vi "movearea_old.vi"(8 "error in (no error)":errorcluster, 11 "Input":string="y-") -> (0 "error out":errorcluster, 3 "Output":string)   [LabVIEW 2014]
uses:
  <userlib>/Nanonis Prog Interface V5/Nanonis Prog Interface.lvlib
panel:
  out "size(s)":i32=3
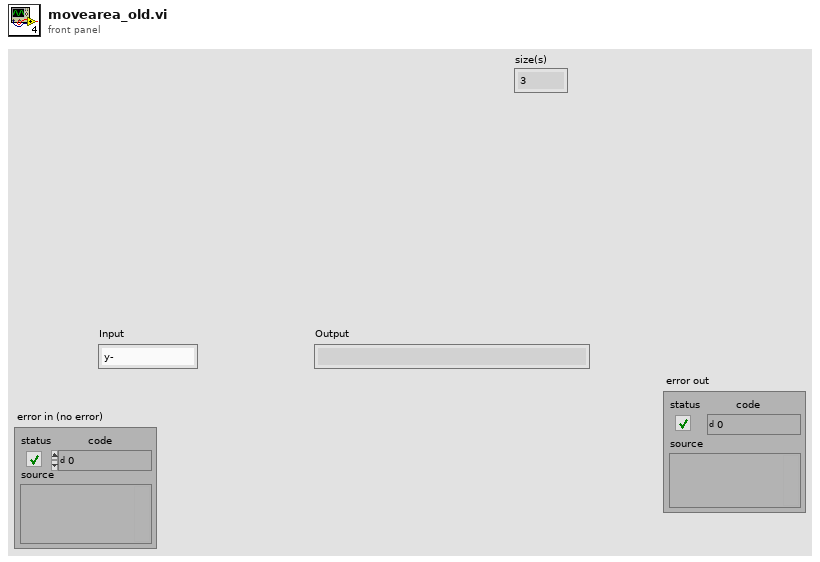
[diagram p1: front panel]
types:
  T1 = enum8{"Group 1", "Group 2", "Group 3", "Group 4", "Group 5", "Group 6"}
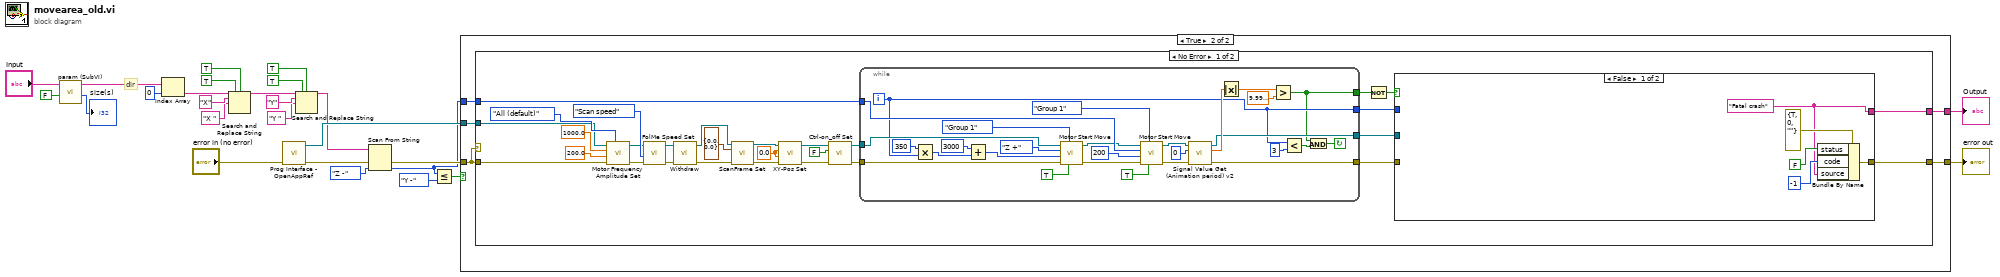
[diagram p0: block diagram]
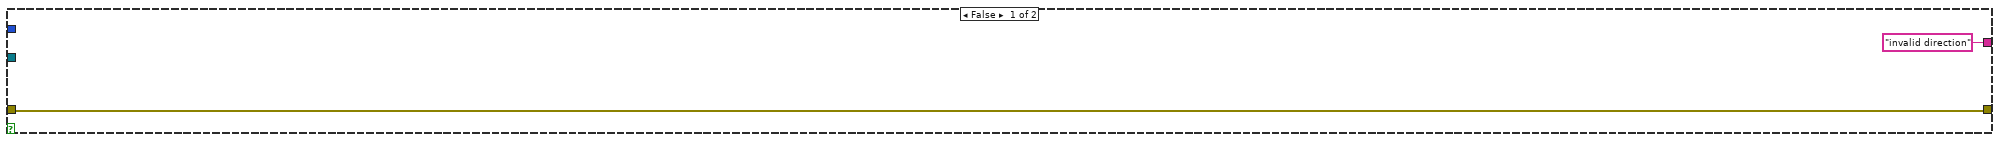
[diagram p2: hidden frame]
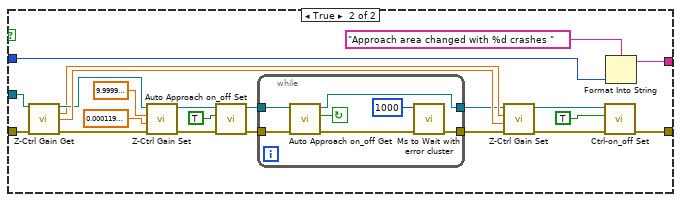
[diagram p3: hidden frame]
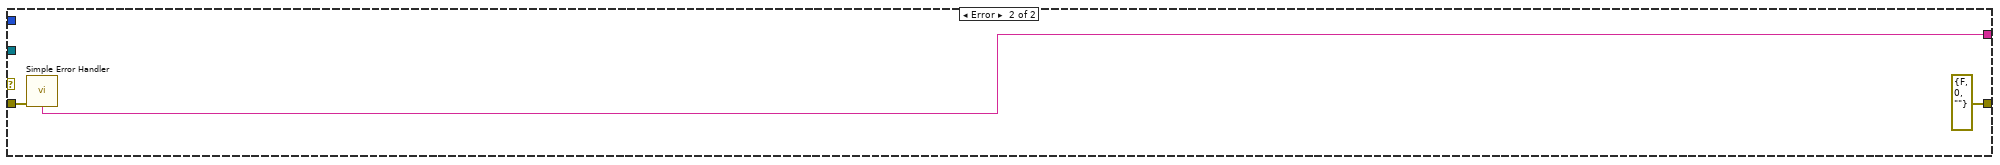
[diagram p4: hidden frame]
diagram:
  # "dir"
  n1 = call <userlib>:"param (SubVI).vi"("Numeric"=FALSE, "Input"="Input") -> ("num"=→"size(s)":i32, "Array"=w22:string[])  [unwired: 7 in, 1 out]
  n2 = Index Array(array=w22, index=0) -> (element=w11:string)
  n3 = Search and Replace String(replace all?=TRUE ("replace all? (F)"), case sensitive?=TRUE ("ignore case? (F)"), input string=w11, search string="X", replace string="X " ("replace string (\"\")")) -> (result string=w2:string)  [unwired: 3 in, 3 out]
  n4 = call <userlib>:"Prog Interface - OpenAppRef.vi"("Error in (no error)"="error in (no error)") -> ("Error out"=w19:errorcluster, "Application reference"=w23:refnum<vi>)  [unwired: 5 in]
  n5 = Search and Replace String(replace all?=TRUE ("replace all? (F)"), case sensitive?=TRUE ("ignore case? (F)"), input string=w2, search string="Y", replace string="Y " ("replace string (\"\")")) -> (result string=w1:string)  [unwired: 3 in, 3 out]
  n6 = Scan From String(input string=w1, error in=w19, default 1=enum16{"X +", "X -", "Y +", "Y -", "Z +", "Z -"}."Z -" ("Direction")) -> (error out=w18:errorcluster, output 1=w15:enum16{"X +", "X -", "Y +", "Y -", "Z +", "Z -"})  [unwired: 2 in, 2 out]
  n7 = Less Or Equal?(x=w15, y=enum16{"X +", "X -", "Y +", "Y -", "Z +", "Z -"}."Y -") -> (x <= y?=w13:bool)
  n8 = case shown="True" w13 {
    tunnel: w23 -> [_ w33]
    tunnel: w15 -> [_ w32]
    tunnel: w18 -> [w28 w31]
    tunnel: [w28 w30] -> w17
    tunnel: ["invalid direction" ("message") w29] -> w16
    frame False {
    }
    frame True {
      n9 = case shown="No Error" w31 {
        tunnel: w33 -> [w50 _]
        tunnel: w32 -> [w48 _]
        tunnel: w31 -> [w47 w127]
        tunnel: [w34 errorcluster {"status"=FALSE, "code"=0, "source"=""} ("error out")] -> w30
        tunnel: [w39 w126] -> w29
        frame No Error {
          w57 = sgl 0.0 ("X (m)")
          n10 = call <userlib>:"Motor Frequency Amplitude Set.vi"("Axis (All)"=enum16{"All (default)", "X", "Y", "Z"}."All (default)", "Error in (no error)"=w47, "Amplitude (V) (NaN=no change)"=sgl 200.0, "Frequency (Hz) (NaN=no change)"=sgl 1000.0, "Application ref in"=w50) -> ("Error out"=w46:errorcluster, "Application ref out"=w49:refnum<vi>)  [unwired: 5 in]
          n11 = call <userlib>:"FolMe Speed Set.vi"("error in (no error)"=w46, "Speed Setting (Custom)"=enum32{"Scan speed", "Custom speed"}."Scan speed", "Application ref in"=w49) -> ("error out"=w54:errorcluster, "Application ref out"=w55:refnum<vi>)  [unwired: 5 in]
          n12 = call <userlib>:"Withdraw.vi"("Error in (no error)"=w54, "Application ref in"=w55) -> ("Error out"=w61:errorcluster, "Application ref out"=w62:refnum<vi>)  [unwired: 8 in]
          n13 = call <userlib>:"ScanFrame Set.vi"("Application ref in"=w62, "Center coordinates (m)"=cluster{"Xc":sgl, "Yc":sgl} {"Xc"=0.0, "Yc"=0.0}, "error in (no error)"=w61) -> ("Application ref out"=w58:refnum<vi>, "error out"=w59:errorcluster)  [unwired: 11 in]
          n14 = call <userlib>:"XY-Pos Set.vi"("error in (no error)"=w59, "Y (m)"=w57, "X (m)"=w57, "Application ref in"=w58) -> ("error out"=w40:errorcluster, "Application ref out"=w41:refnum<vi>)  [unwired: 4 in]
          n15 = call <userlib>:"Ctrl-on_off Set.vi"("error in (no error)"=w40, "Z Controller ON/OFF"=FALSE, "Application ref in"=w41) -> ("error out"=w42:errorcluster, "Application ref out"=w43:refnum<vi>)  [unwired: 7 in]
          n16 = while {
            tunnel: w48 -> [w124]
            tunnel: [w102] -> w45
            tunnel: [w101] -> w44
            tunnel: w43 -> [w100]
            tunnel: w42 -> [w99]
            tunnel: [w98] -> w38
            tunnel: [w97] -> w37
            i -> [w98]
            stop <- w104 continue-if-true
            n17 = Multiply(x=350, y=w98) -> (x*y=w107:i32)
            n18 = Add(x=u16 3000 ("Number of steps"), y=w107) -> (x+y=w109:i32)
            n19 = call <userlib>:"Motor Start Move.vi"("Wait until finished? (F)"=TRUE, "Group"=T1."Group 1", "Error in (no error)"=w99, "Number of steps"=w109, "Direction"=enum16{"X +", "X -", "Y +", "Y -", "Z +", "Z -"}."Z +", "Application ref in"=w100) -> ("Error out"=w119:errorcluster, "Application ref out"=w120:refnum<vi>)  [unwired: 3 in]
            n20 = call <userlib>:"Motor Start Move.vi"("Wait until finished? (F)"=TRUE, "Group"=T1."Group 1", "Error in (no error)"=w119, "Number of steps"=u16 200, "Direction"=w124, "Application ref in"=w120) -> ("Error out"=w113:errorcluster, "Application ref out"=w115:refnum<vi>)  [unwired: 3 in]
            n21 = call <userlib>:"Signal Value Get (Animation period) v2.vi"("error in (no error)"=w113, "Signal index (0-79)"=i8 0, "Application ref in"=w115) -> ("error out"=w101:errorcluster, "Signal value"=w112:sgl, "Application ref out"=w102:refnum<vi>)  [unwired: 5 in]
            n22 = Absolute Value(x=w112) -> (abs(x)=w110:sgl)
            n23 = Greater?(x=w110, y=sgl 1e-09) -> (0:w97:bool)
            n24 = Less?(x=w98, y=3) -> (x < y?=w103:bool)
            n25 = And(x=w97, y=w103) -> (x .and. y?=w104:bool)
          }
          n26 = Not(x=w37) -> (.not. x?=w36:bool)
          n27 = case shown="False" w36 {
            tunnel: w45 -> [_ w89]
            tunnel: w44 -> [_ w79]
            tunnel: [w64 w71] -> w39
            tunnel: w38 -> [_ w70]
            tunnel: [w63 w68] -> w34
            frame False {
              w64 = "Fatal crash"
              n28 = Bundle By Name(cluster=errorcluster {"status"=TRUE, "code"=0, "source"=""} ("error out"), "status"=FALSE, "code"=-1, "source"=w64) -> (w63:errorcluster)
            }
            frame True {
              n29 = call <userlib>:"Z-Ctrl Gain Get.vi"("Application ref in"=w89, "error in (no error)"=w79) -> ("Application ref out"=w85:refnum<vi>, "P-gain"=w83:sgl, "Time constant (s)"=w88:sgl, "error out"=w78:errorcluster)  [unwired: 9 in, 1 out]
              n30 = call <userlib>:"Z-Ctrl Gain Set.vi"("error in (no error)"=w78, "Time constant (s)"=sgl 0.00012, "P-gain"=sgl 1e-11, "Application ref in"=w85) -> ("error out"=w77:errorcluster, "Application ref out"=w84:refnum<vi>)  [unwired: 5 in]
              n31 = call <userlib>:"Auto Approach on_off Set.vi"("Error in (no error)"=w77, "Auto approach start/stop (F)"=TRUE, "Application ref in"=w84) -> ("Error out"=w76:errorcluster, "Application ref out"=w81:refnum<vi>)  [unwired: 5 in]
              n32 = while {
                tunnel: w81 -> [w93]
                tunnel: [w92] -> w80
                tunnel: w76 -> [w91]
                tunnel: [w90] -> w75
                stop <- w96 continue-if-true
                n33 = call <userlib>:"Auto Approach on_off Get.vi"("Error in (no error)"=w91, "Application ref in"=w93) -> ("Error out"=w94:errorcluster, "Auto approach on/off status"=w96:bool, "Application ref out"=w92:refnum<vi>)  [unwired: 5 in]
                n34 = call <userlib>:"Ms to Wait with error cluster.vi"("error in (no error)"=w94, "milliseconds to wait"=u32 1000) -> ("error out"=w90:errorcluster)  [unwired: 4 in, 1 out]
              }
              n35 = call <userlib>:"Z-Ctrl Gain Set.vi"("error in (no error)"=w75, "Time constant (s)"=w88, "P-gain"=w83, "Application ref in"=w80) -> ("error out"=w72:errorcluster, "Application ref out"=w74:refnum<vi>)  [unwired: 5 in]
              n36 = call <userlib>:"Ctrl-on_off Set.vi"("error in (no error)"=w72, "Z Controller ON/OFF"=TRUE, "Application ref in"=w74) -> ("error out"=w68:errorcluster)  [unwired: 7 in, 1 out]
              n37 = Format Into String(format string="Approach area changed with %d crashes " ("initial string"), w70) -> (resulting string=w71:string)  [unwired: 2 in, 1 out]
            }
          }
        }
        frame Error {
          n38 = call <vilib>:"Simple Error Handler.vi"("error in (no error)"=w127) -> ("message"=w126:string)  [unwired: 4 in, 4 out]
        }
      }
    }
  }
  "Output" <- w16
  "error out" <- w17
